vi "Abort Plugin.vi"(6 "timeout (ms)":i32=5000, 8 "error in":errorcluster, 10 "plugin_name":string, 11 "gRPC ID in":T1) -> (0 "error out":errorcluster, 3 "gRPC ID out":T1)   [LabVIEW 2021, in "CIFPluginLoaderClientWrapper.lvlib"]
uses:
  CIFPluginLoaderClientWrapper.lvlib
  CIF_PluginLoader_client/CIF_PluginLoader_client.lvlib
  CIF_PluginLoader_client/RPC Messages/cif_manager_PluginName.ctl
  CIF_PluginLoader_client/RPC Messages/cif_pluginloader_AbortPluginRequest.ctl
  <vilib>/gRPC/LabVIEW gRPC Library/Shared/grpcId.ctl
  <vilib>/gRPC/LabVIEW gRPC Library/grpc-lvsupport-release.lvlib
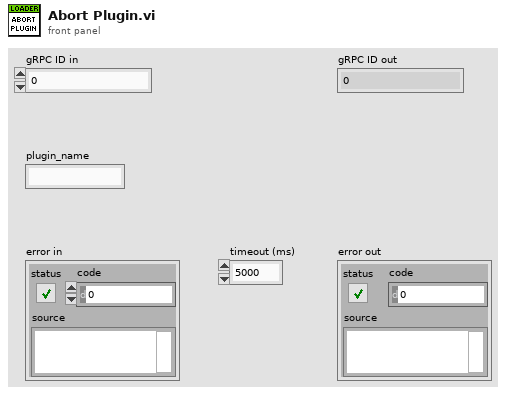
[diagram p1: front panel]
types:
  T1 = typedef "grpc-lvsupport-release.lvlib/grpcId.ctl" = u64
  T2 = typedef "CIF_PluginLoader_client.lvlib/cif_pluginloader_AbortPluginRequest.ctl" = cluster{"plugin_name":T3}
  T3 = typedef "CIF_PluginLoader_client.lvlib/cif_manager_PluginName.ctl" = cluster{"plugin_name":string}
  T4 = typedef "CIF_PluginLoader_client.lvlib/cif_pluginloader_AbortPluginResponse.ctl" = cluster{"status":T5}
  T5 = typedef "CIF_PluginLoader_client.lvlib/cif_common_Status.ctl" = cluster{"code":i32, "message":string}
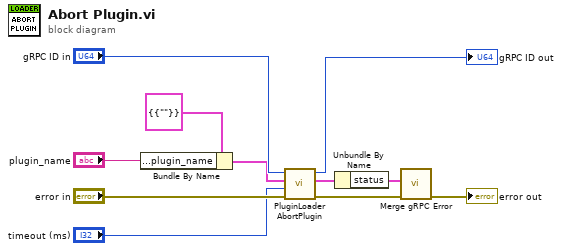
[diagram p0: block diagram]
diagram:
  n1 = Bundle By Name(cluster=T2 {"plugin_name"={"plugin_name"=""}} ("Request Data"), "plugin_name.plugin_name"="plugin_name") -> (w3:T2)
  n2 = call "PluginLoader AbortPlugin.vi"("error in"="error in", "timeout (ms)"="timeout (ms)", "Request Data"=w3, "gRPC ID"="gRPC ID in") -> ("error out"=w7:errorcluster, "Response Data"=w5:T4, "gRPC ID out"=→"gRPC ID out":T1)  [unwired: 5 in]
  n3 = Unbundle By Name(w5) -> ("status"=w1:T5)
  n4 = call "Merge gRPC Error.vi"("error in (no error)"=w7, "gRPC Error"=w1) -> ("error out"=→"error out":errorcluster)  [unwired: 9 in]
